vi "ResultsDB Select Record List.vi"() -> (0 "error out":errorcluster, 2 "Row Num List":string[](array[string]), 3 "Table Control":string[][](table))   [LabVIEW 2021, in "SQLite.lvclass"]
doc: "开始测试时根据条目自动创建条目条目，生产文件路径。\n#2020-6-8 13:25:45"
uses:
  SQLite.lvclass
  <vilib>/Utility/error.llb/Trim Whitespace.vi
  SQLite.lvclass/SQLite.ctl
  <userlib>/sushu/sushu.lvlib
  <userlib>/LabSQL/LabSQL.lvlib
  vi.lib_New/TopPath/TopPath.lvlib
panel:
  out "CMD":string
  out "number (0 to 1)":dbl
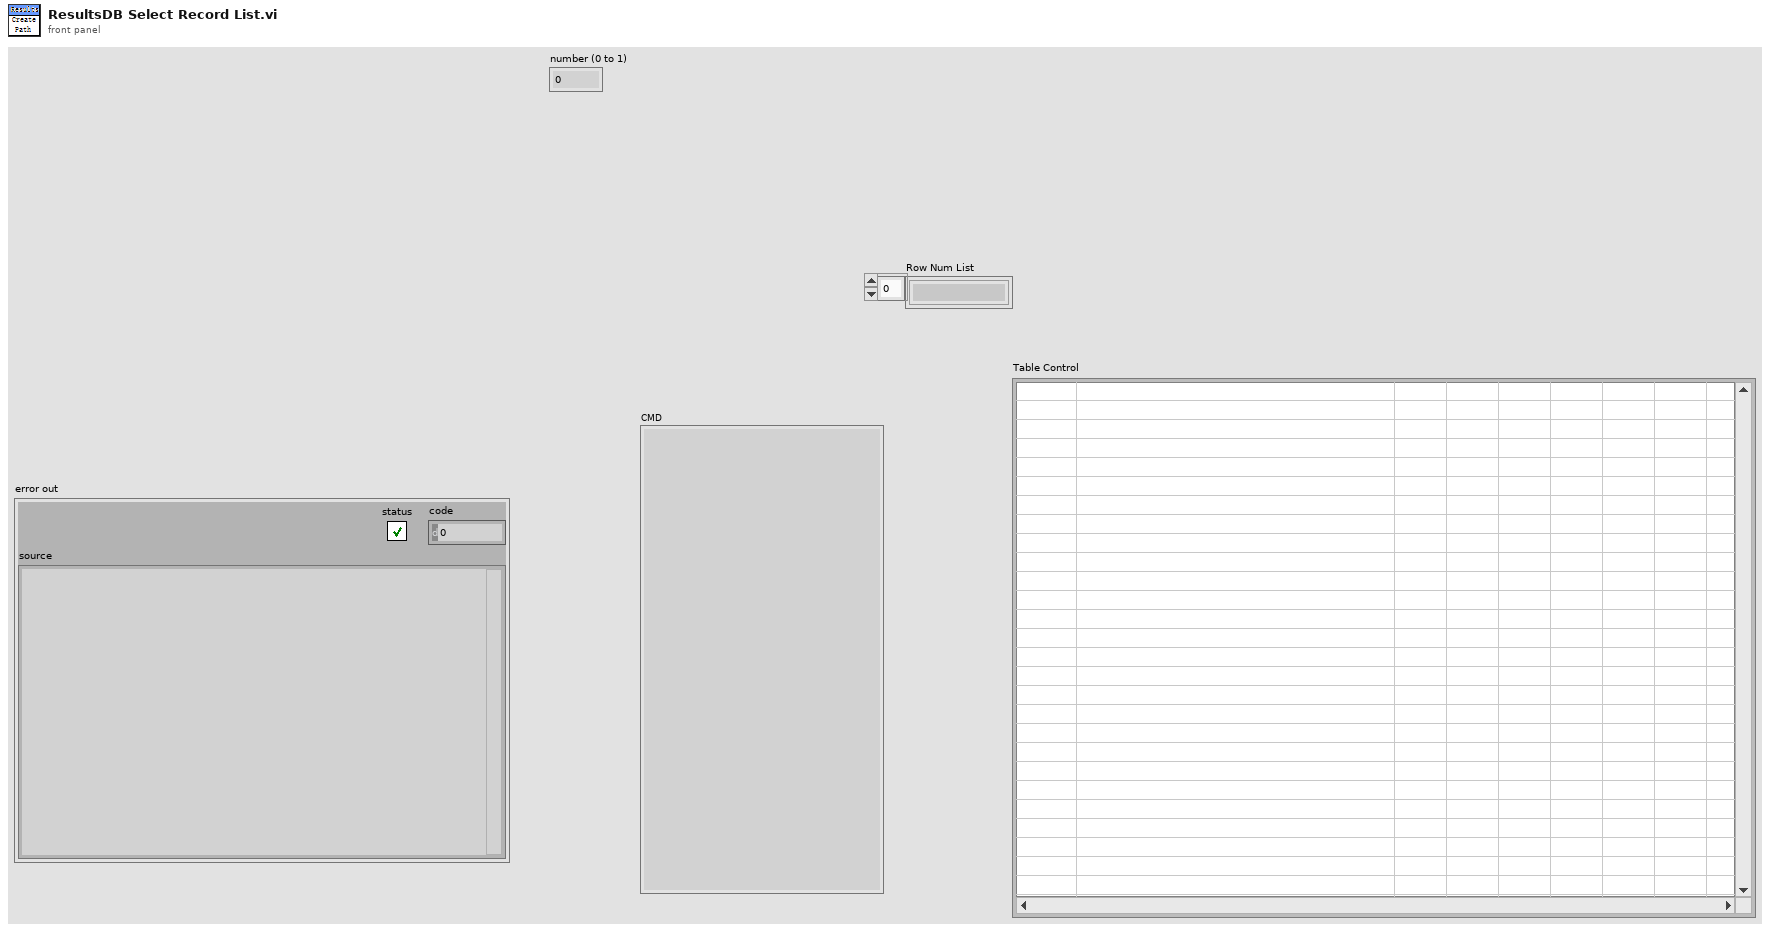
[diagram p1: front panel]
types:
  T1 = cluster{"Core":cluster{"Current VI Reference":refnum<vi>, "Close Panel on Exit?":bool}, "VI Name":string, "Row Numbers":string, "Update?":bool, "Results Folder path":path, "CMD":string, "RowNum":i32, "ResultFilePath":path, "InsertTimes":i32, "length":i32}
  T2 = enum16{"Other", "SQL2008", "SQLite", "Access", "MySQL"}
  T3 = typedef "TopPath.lvlib/Top Path.ctl" = cluster{"LV Source":path, "FilePath":path, "Data":path}
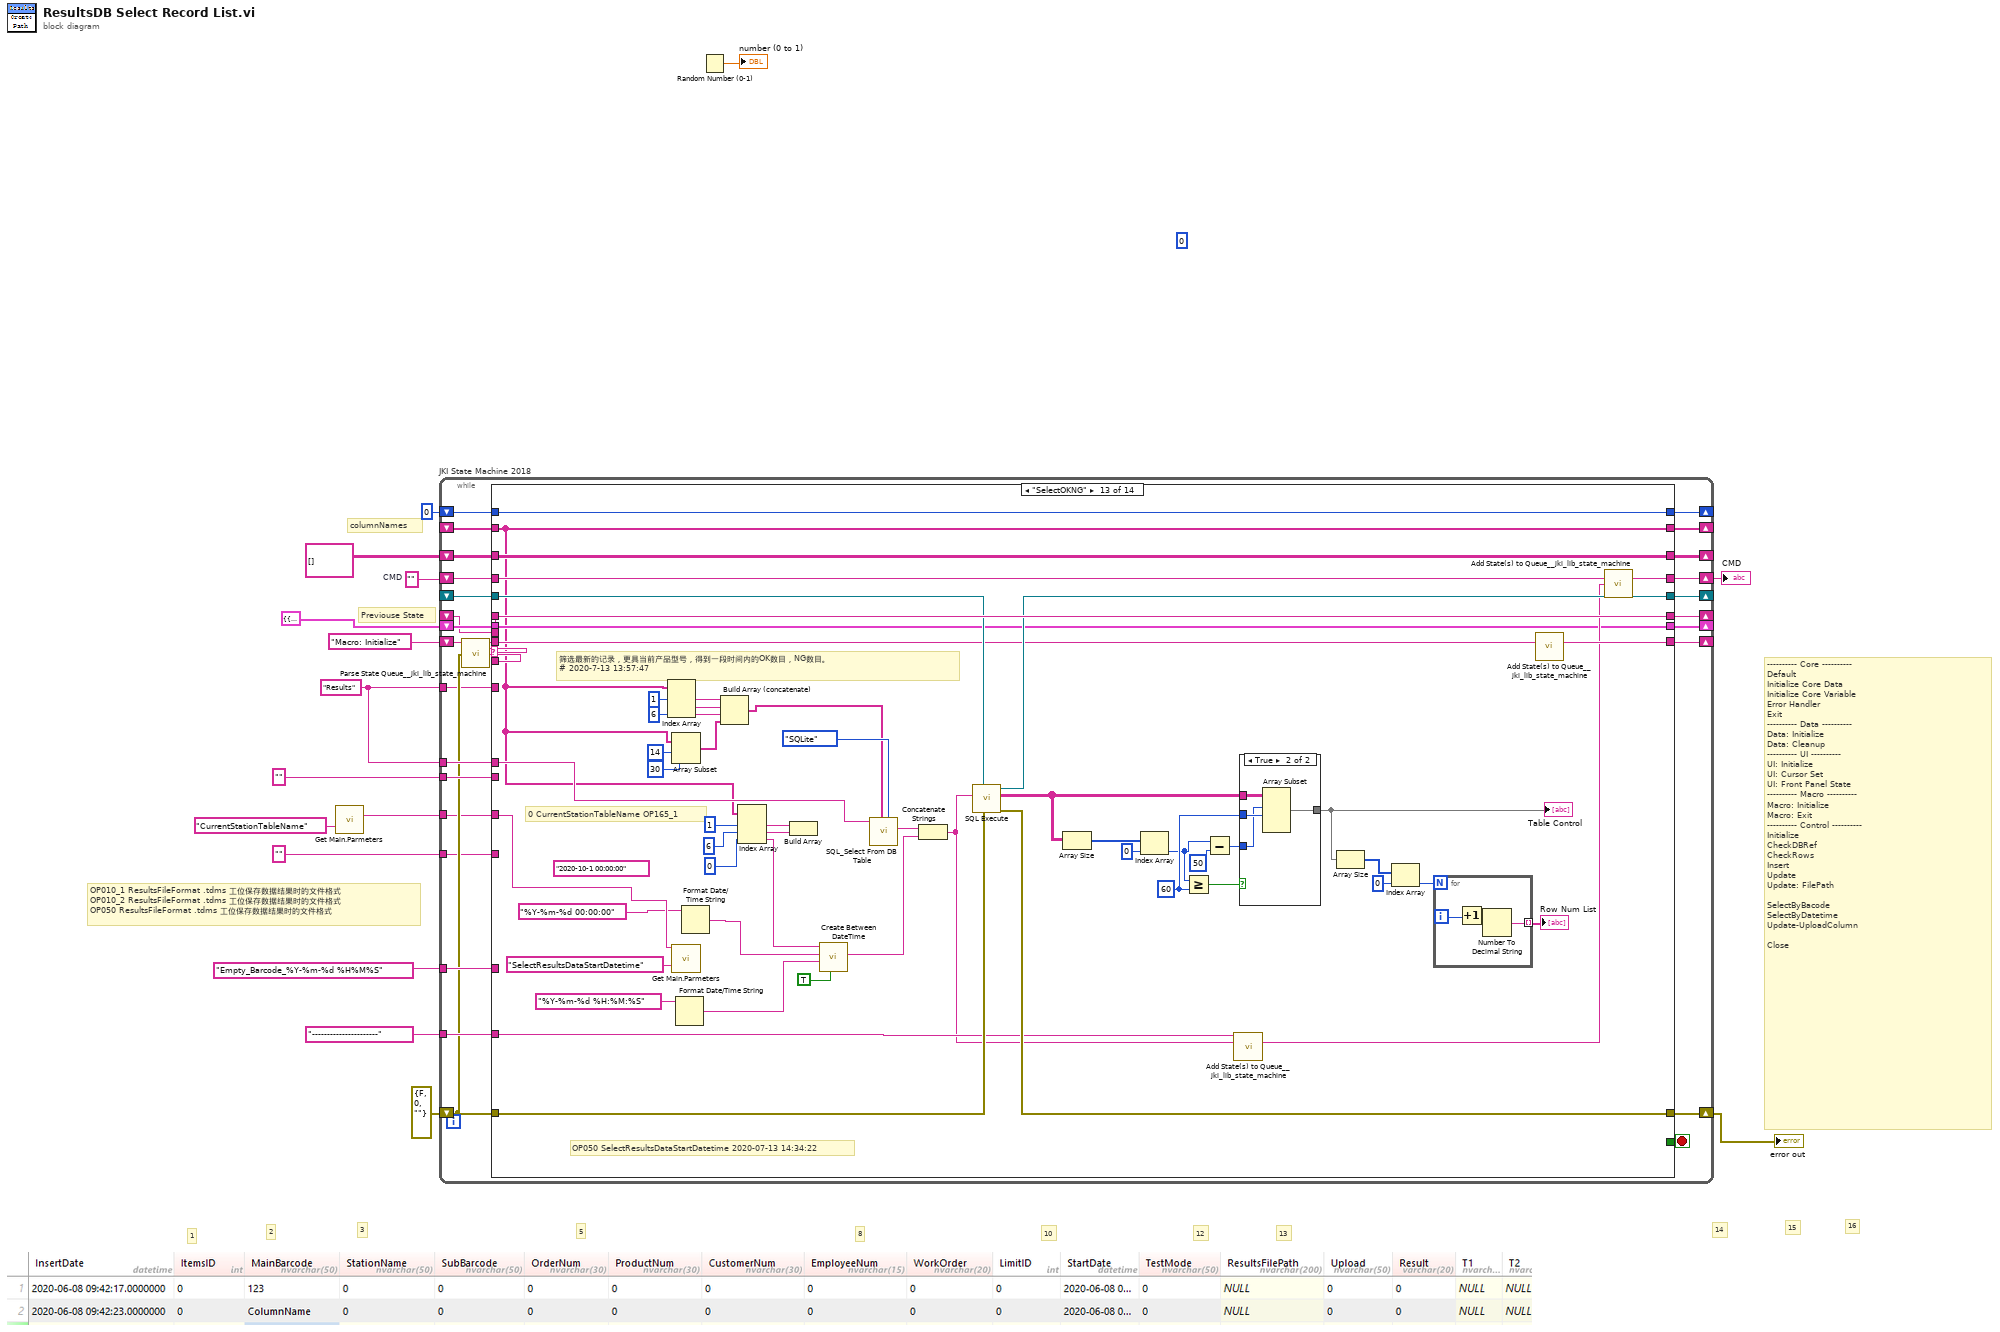
[diagram p0: block diagram]
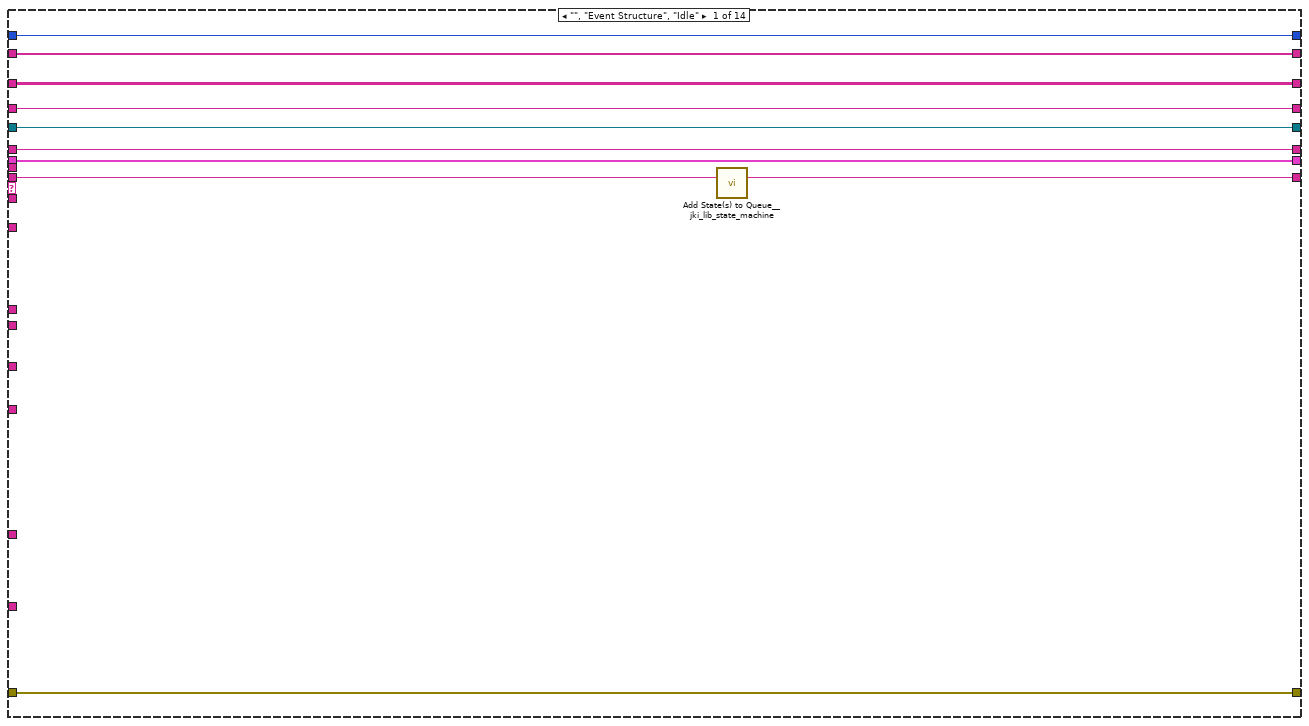
[diagram p2: hidden frame]
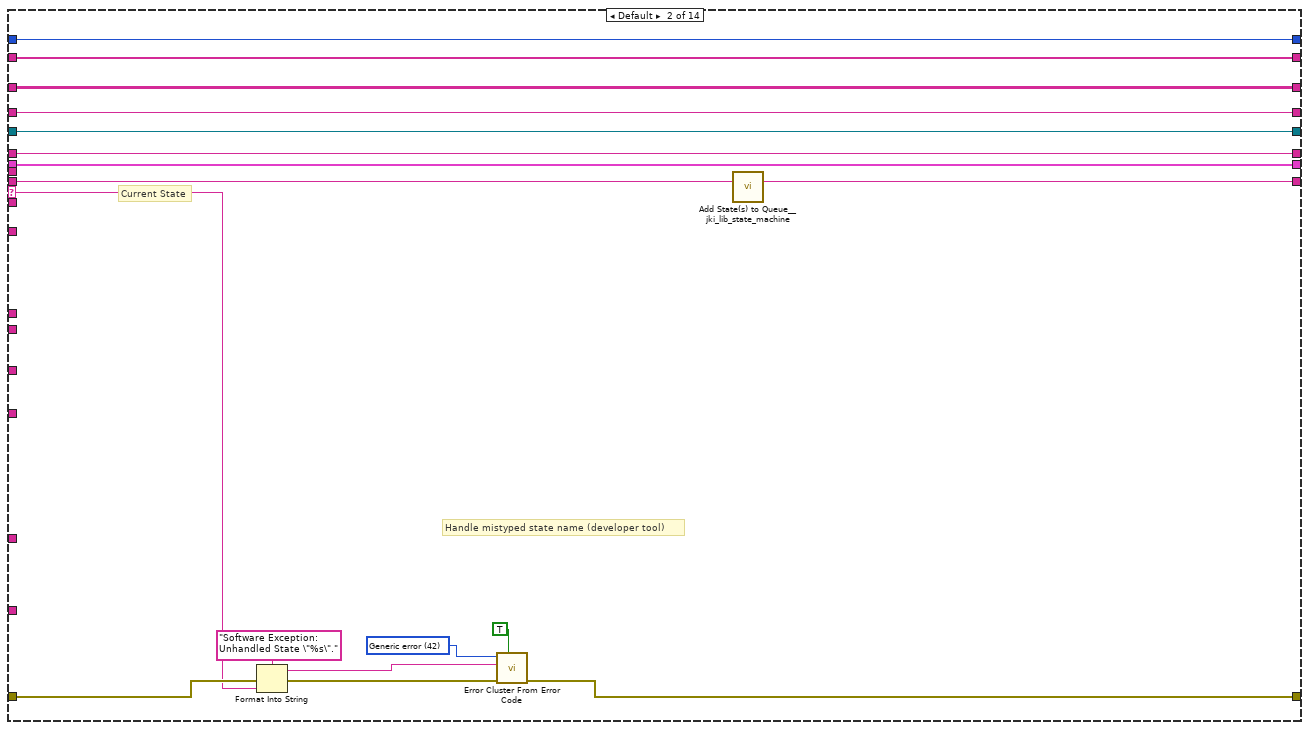
[diagram p3: hidden frame]
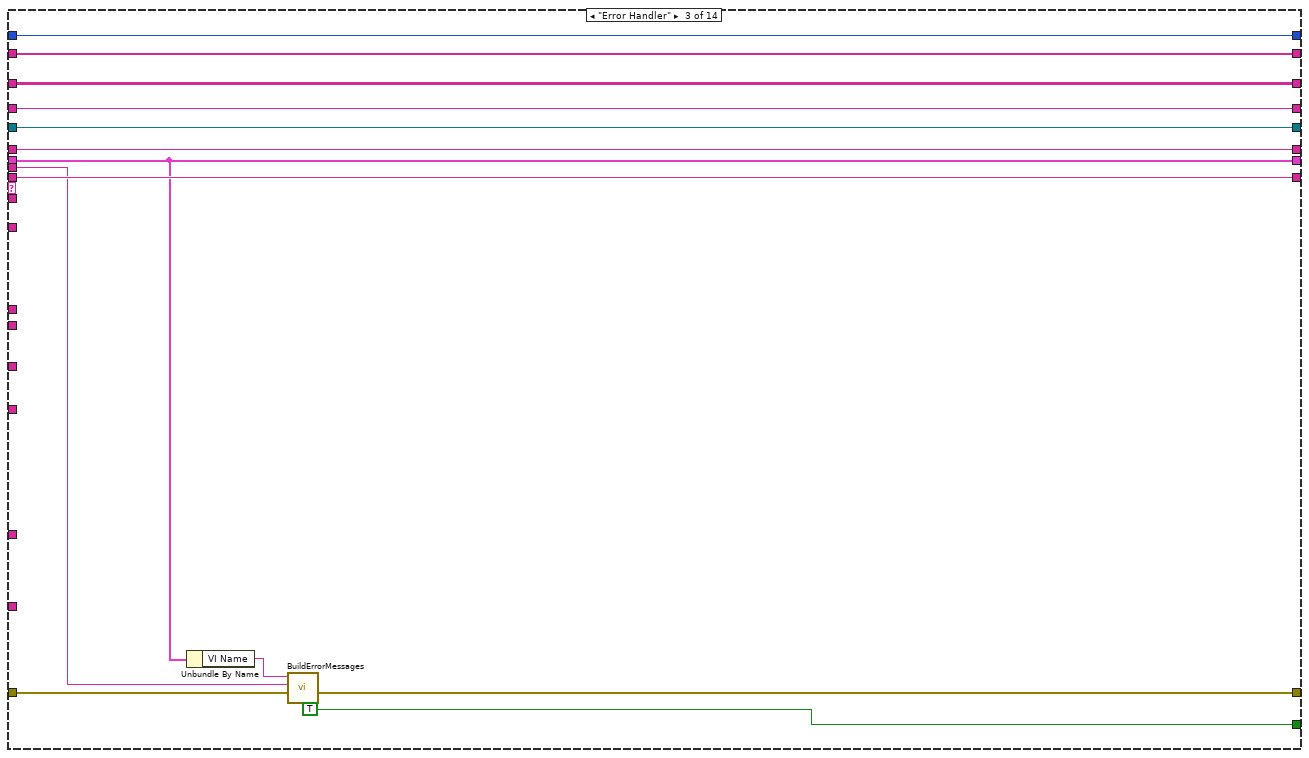
[diagram p4: hidden frame]
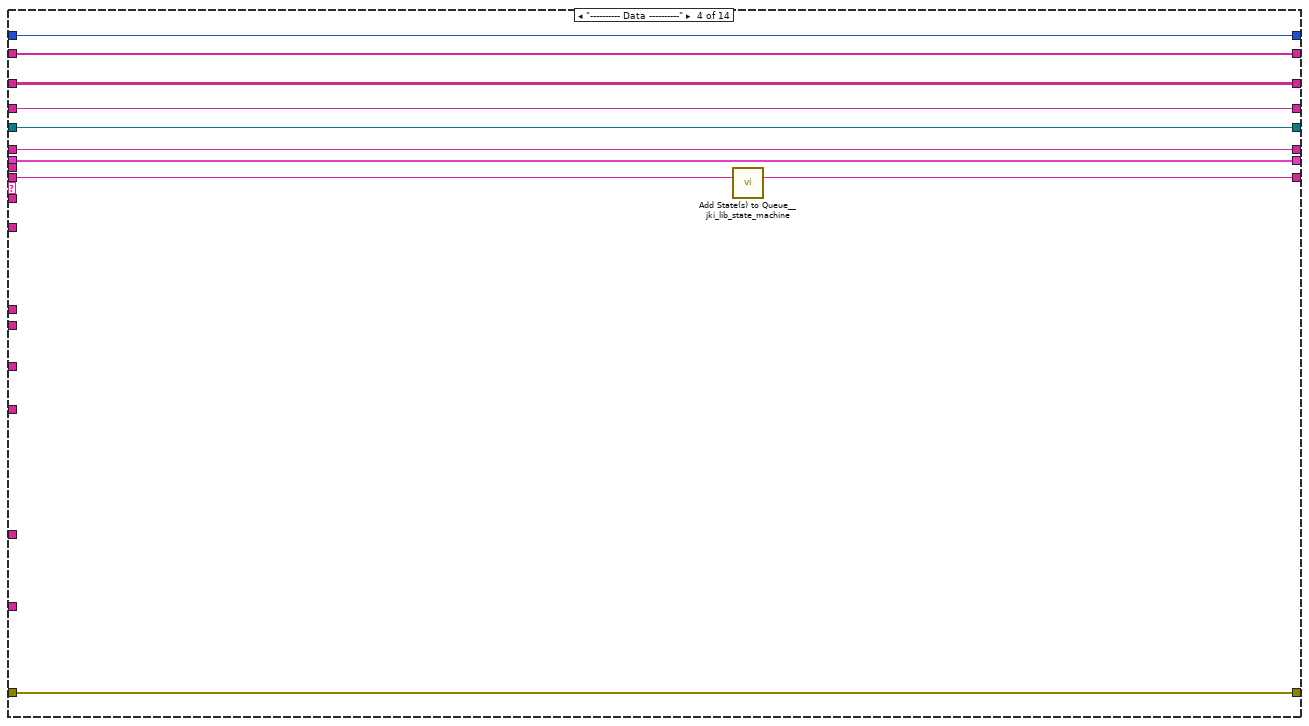
[diagram p5: hidden frame]
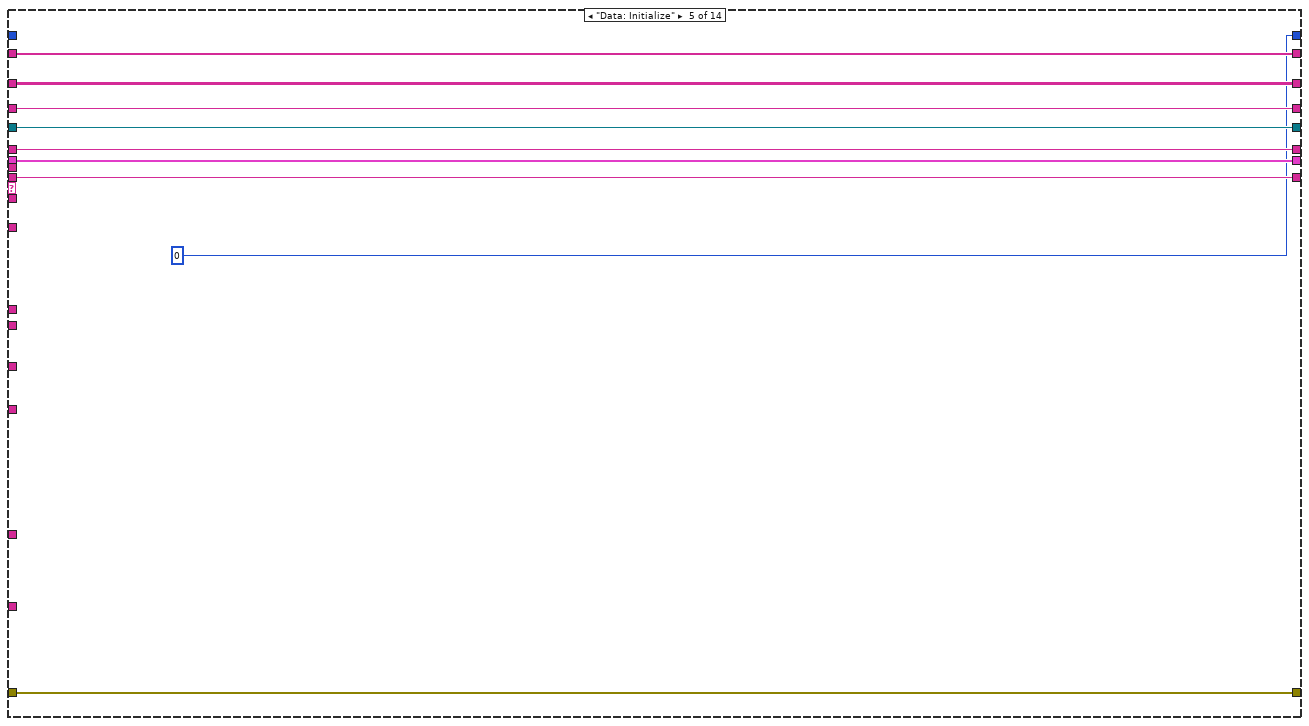
[diagram p6: hidden frame]
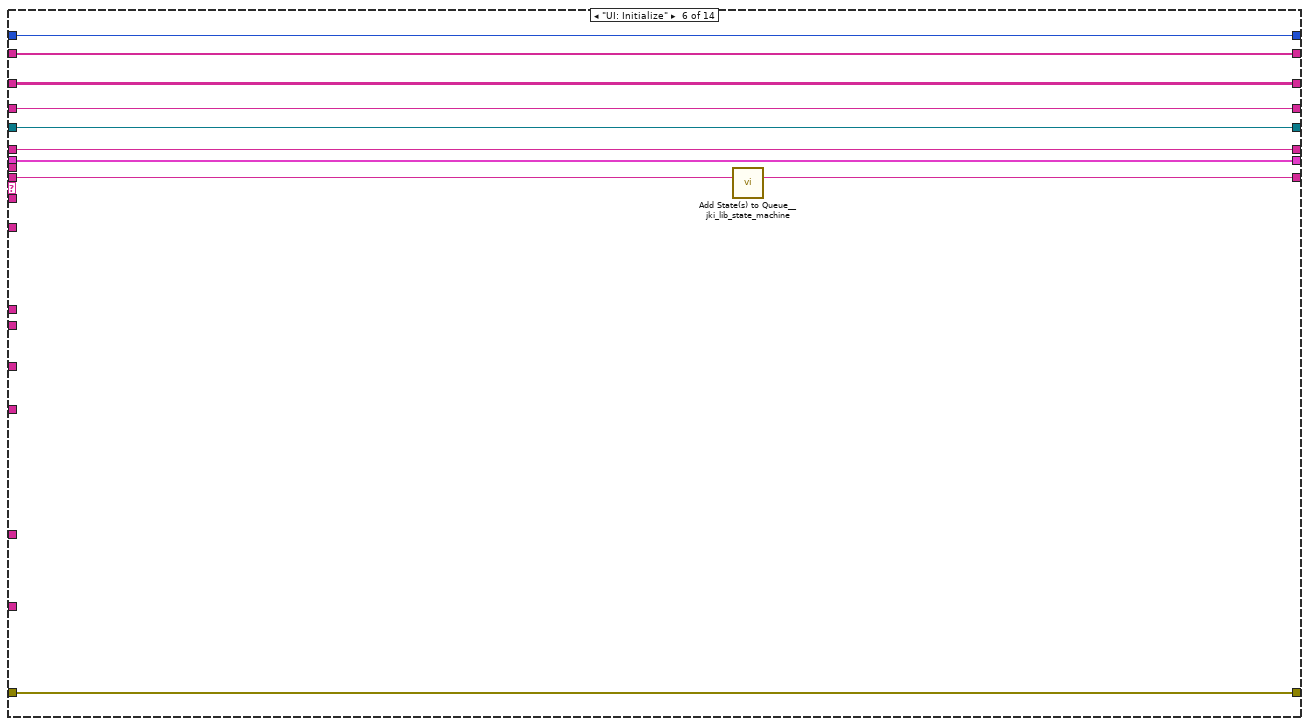
[diagram p7: hidden frame]
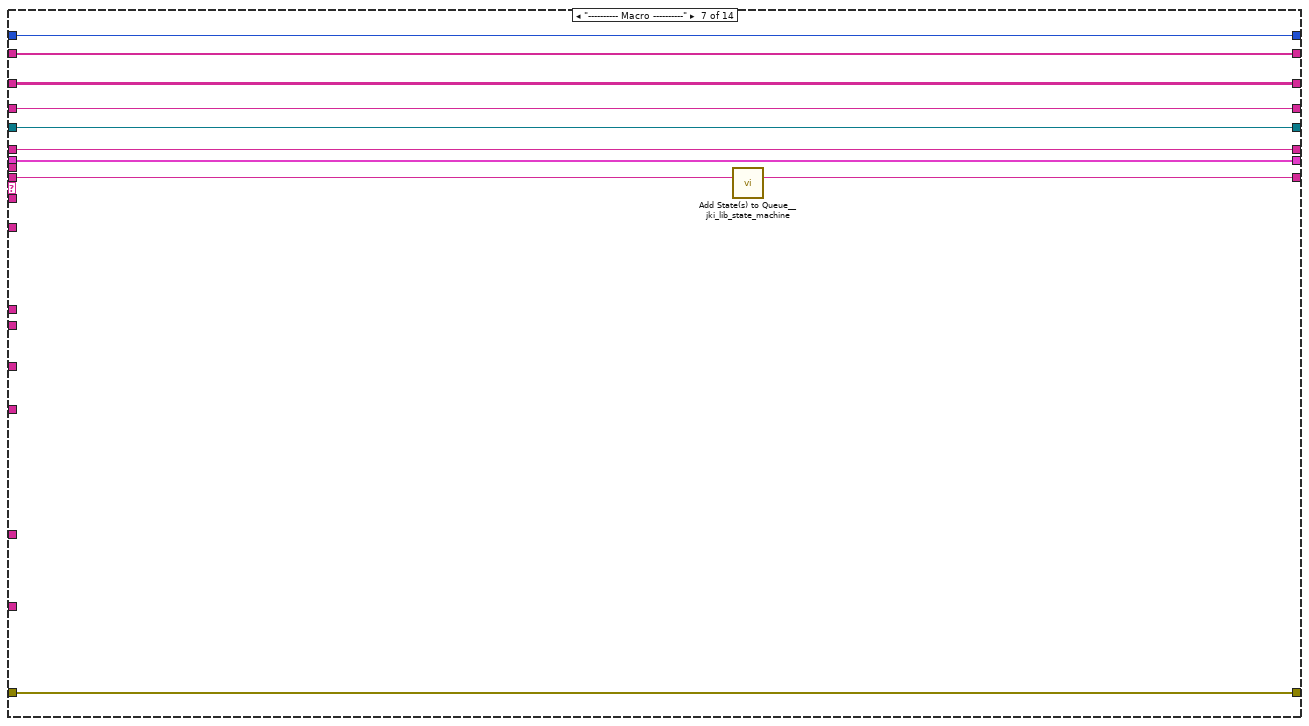
[diagram p8: hidden frame]
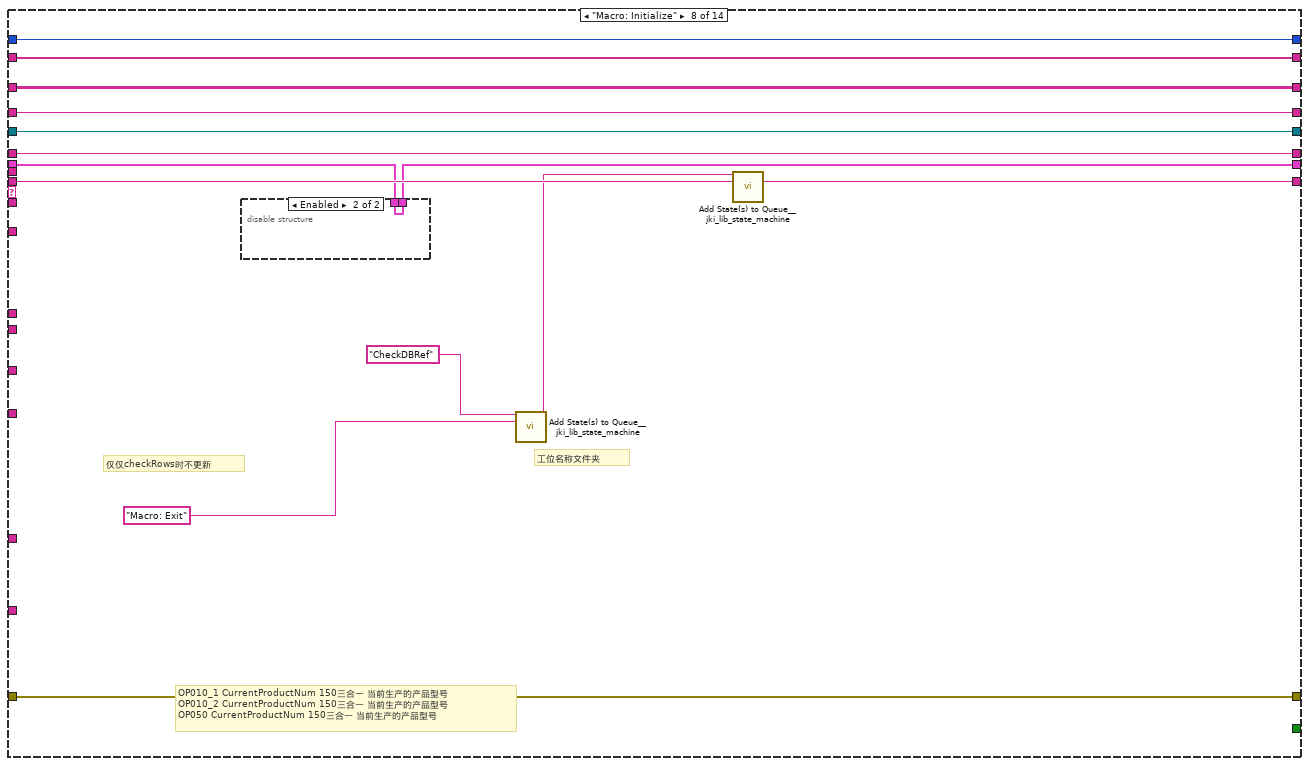
[diagram p9: hidden frame]
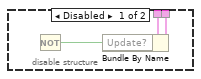
[diagram p10: hidden frame]
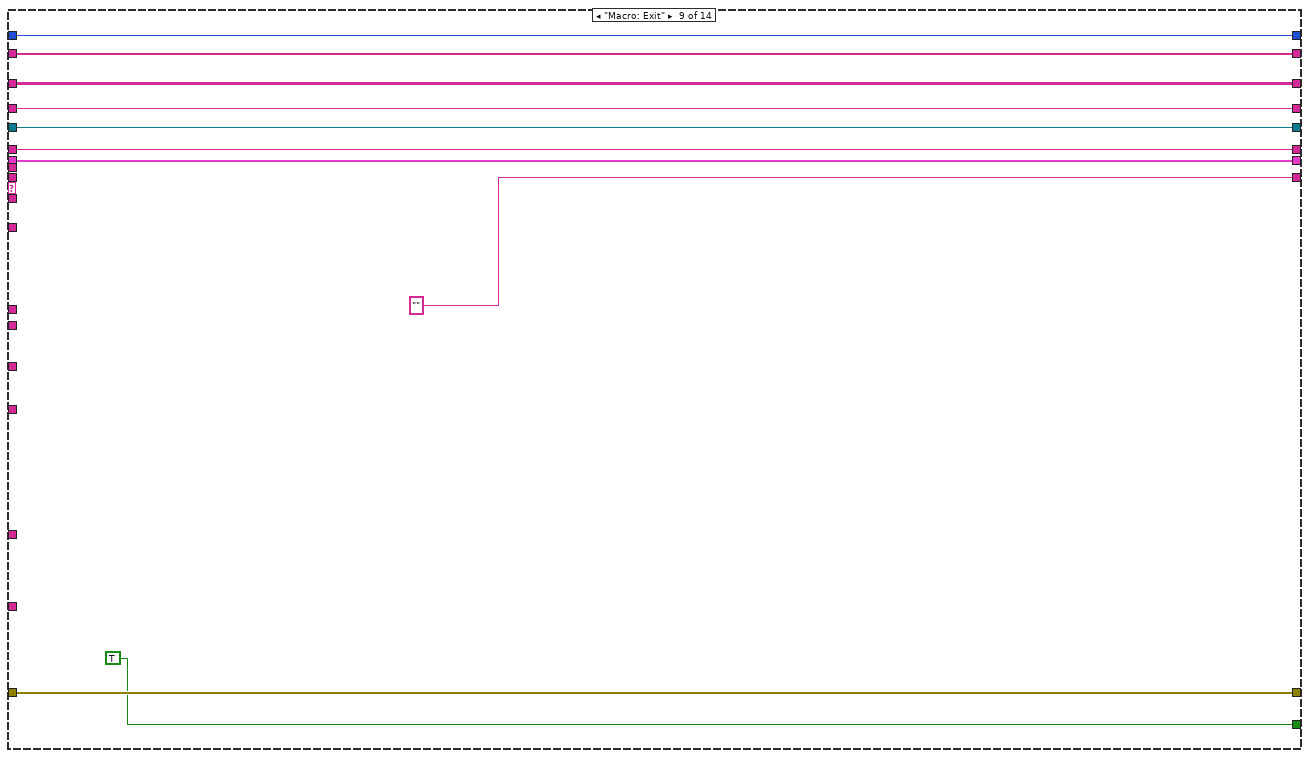
[diagram p11: hidden frame]
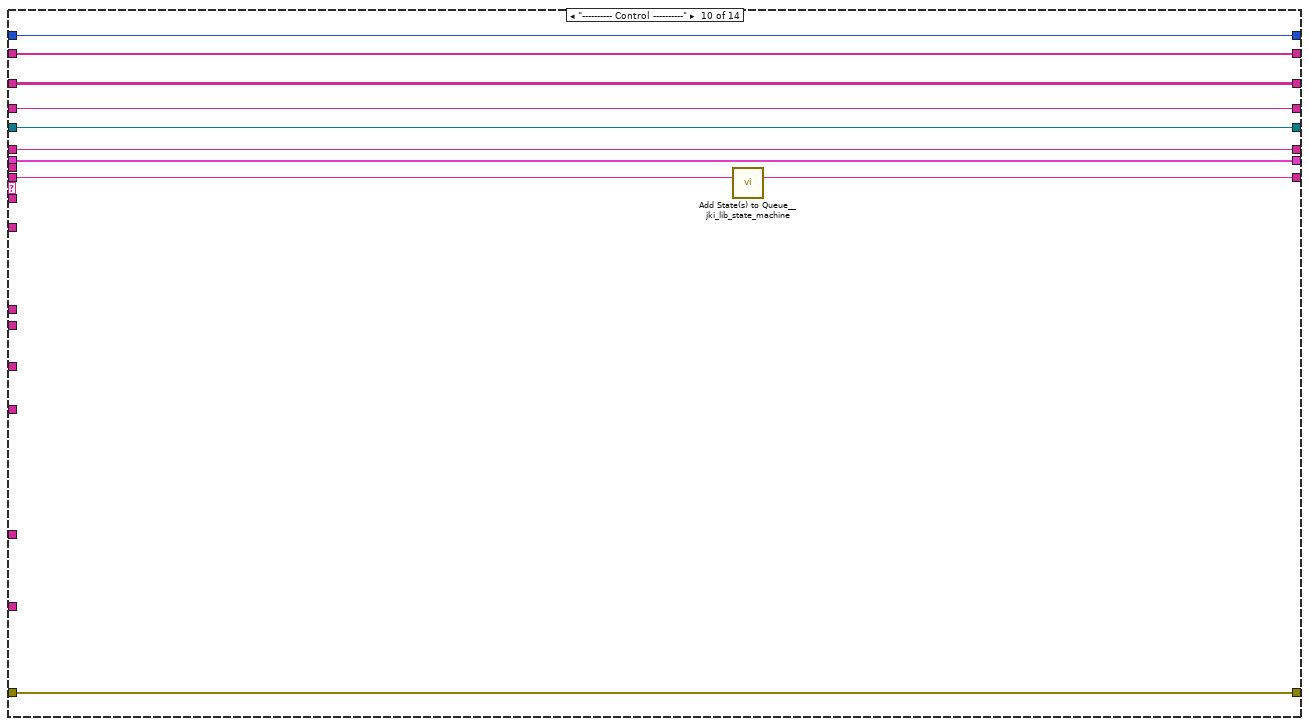
[diagram p12: hidden frame]
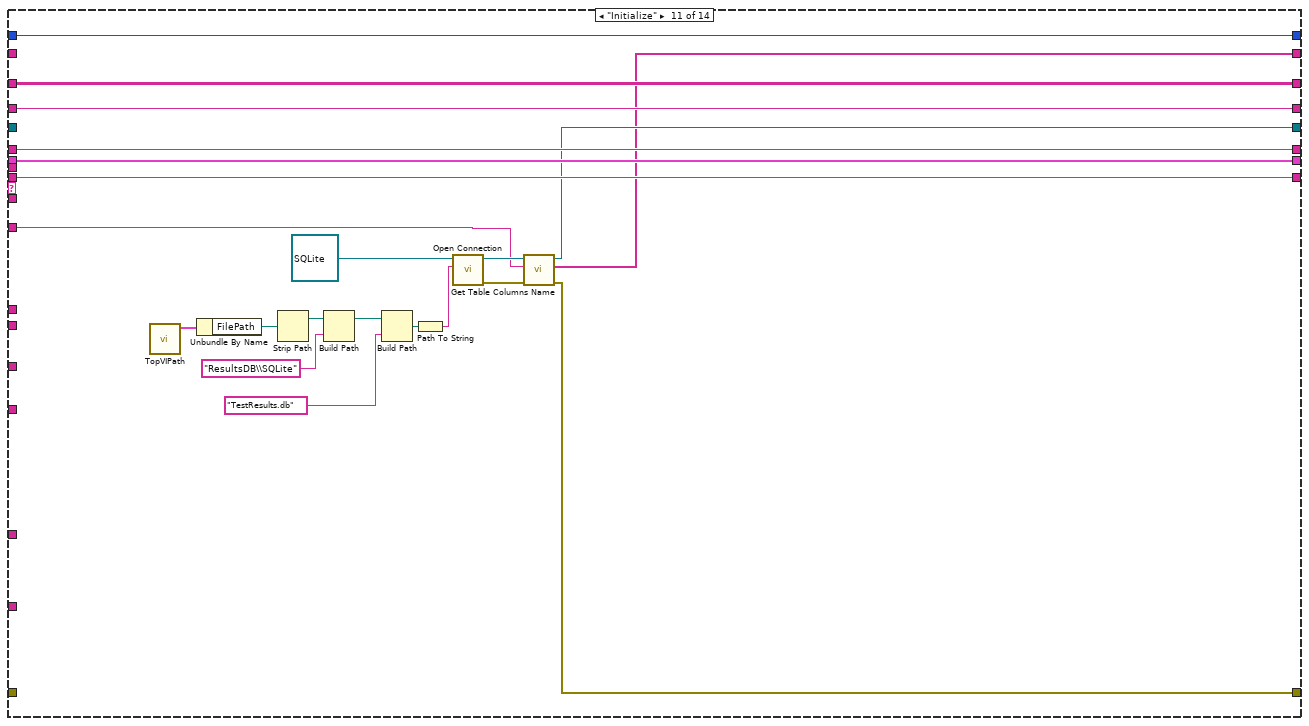
[diagram p13: hidden frame]
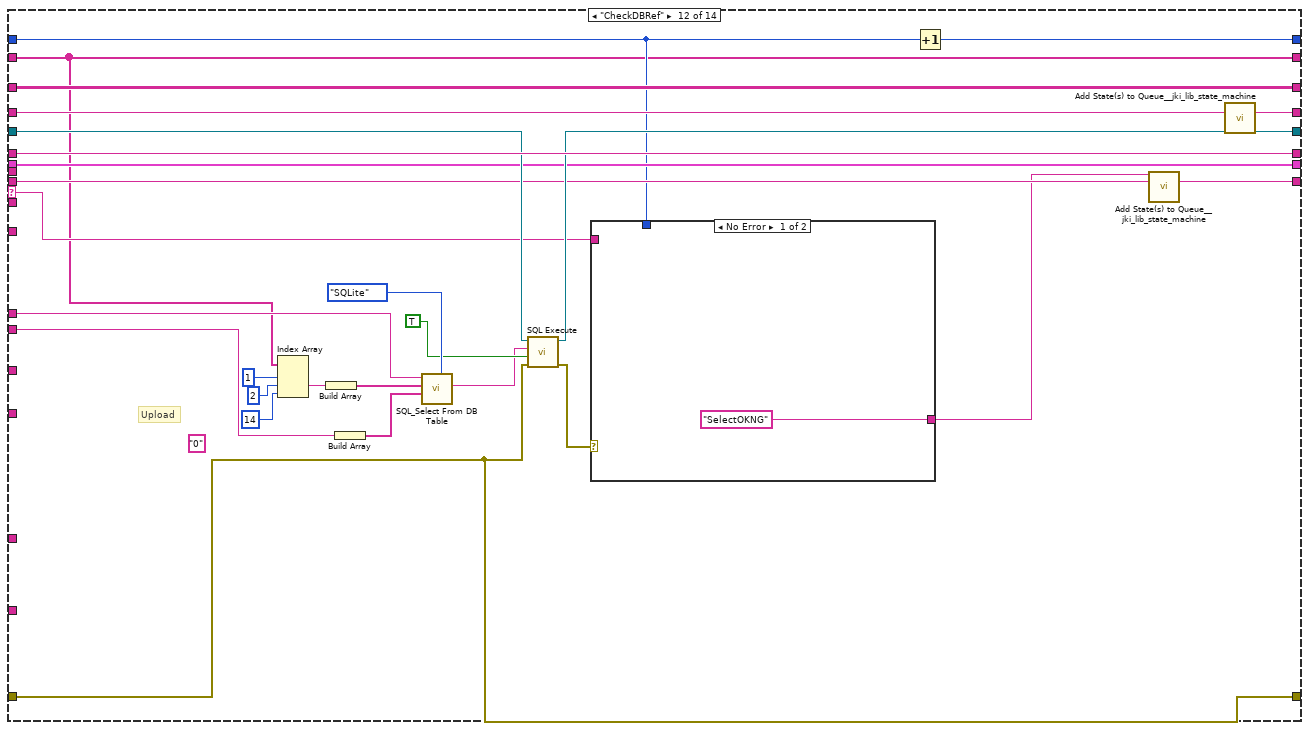
[diagram p14: hidden frame]
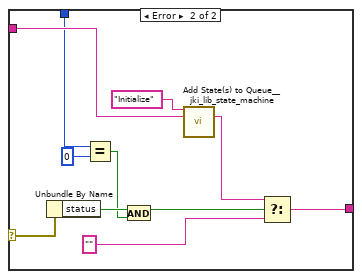
[diagram p15: hidden frame]
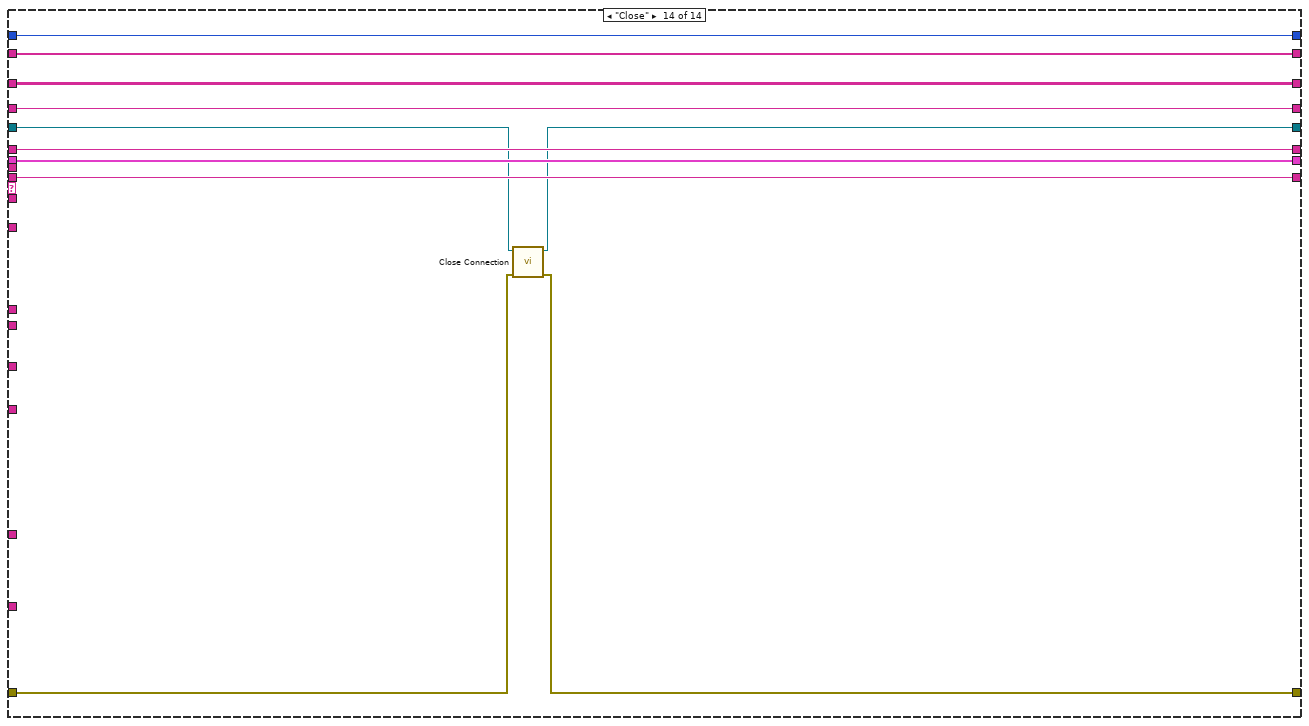
[diagram p17: hidden frame]
diagram:
  w7 = "Results" ("TableName")
  w9 = ""  # CMD
  (unwired) 0 ("index (row)")
  # "columnNames"
  # "OP010_1\tResultsFileFormat\t.tdms\t工位保存数据结果时的文件格式\nOP010_2\tResultsFileFormat\t.tdms\t工位保存数据结果时的文件格式\nOP050\tResultsFileFormat\t.tdms\t工位保存数据结果时的文件格式"
  # "16"
  # "15"
  # "14"
  # "13"
  # "12"
  # "10"
  # "8"
  # "5"
  # "3"
  # "2"
  # "1"
  # "Previouse State"
  # "---------- Core ----------\nDefault\nInitialize Core Data\nInitialize Core Variable\nError Handler\nExit\n---------- Data ----------\nData: Initialize\nData: Cleanup\n---------- UI ----------\nUI: Initialize\nUI: Cursor Set\nUI: Front Panel State\n---------- Macro ----------\nMacro: Initialize\nMacro: Exit\n---------- Control ----------\nInitialize\nCheckDBRef\nCheckRows\nInsert\nUpdate\nUpdate: FilePath\n\nSelectByBacode\nSelectByDatetime\nUpdate-UploadColumn\n\nClose"
  n1 = call "Get Main.Parmeters.vi"("VariableName"="CurrentStationTableName") -> ("Value"=w1:string)  [unwired: 7 in, 7 out]
  n2 = while "JKI State Machine 2018" {
    shift-right: [w39] -> _
    shift-left: T1 {"Core"={"Current VI Reference"=refnum, "Close Panel on Exit?"=FALSE}, "VI Name"="", "Row Numbers"="", "Update?"=FALSE, "Results Folder path"=path "", "CMD"="", "RowNum"=0, "ResultFilePath"=path "", "InsertTimes"=0, "length"=3} ("Data") -> [w38]
    shift-right: [w42] -> w4
    shift-left: errorcluster {"status"=FALSE, "code"=0, "source"=""} ("error out") -> [w24]
    shift-right: [w41] -> _
    shift-left: "Macro: Initialize" -> [w43]
    shift-right: [w36] -> _
    shift-left: _ -> [w37]
    shift-right: [w34] -> _
    shift-left: _ -> [w33]
    tunnel: "" ("MainBarcode") -> [w32]
    tunnel: w7 -> [w31]
    tunnel: "Empty_Barcode_%Y-%m-%d %H%M%S" ("time format string (%c)") -> [w30]
    shift-right: [w29] -> w3
    shift-left: w9 -> [w28]
    tunnel: "----------------------" ("State(s) in (\"\")") -> [w27]
    shift-right: [w25] -> _
    shift-left: string[][] [] ("Table Control") -> [w26]
    tunnel: "" ("ItemsID") -> [w23]
    tunnel: w7 -> [w22]
    shift-right: [w21] -> _
    shift-left: _ -> [w20]
    shift-right: [w18] -> _
    shift-left: 0 -> [w19]
    tunnel: w1 -> [w17]
    stop <- w40 stop-if-true
    n3 = call <vilib>:"Parse State Queue__jki_lib_state_machine.vi"("State Queue"=w43, "Error In (no error)"=w24) -> ("Remaining States"=w45:string, "Current State"=w35:string, "Arguments"=w44:string)  [unwired: 10 in, 1 out]
    n4 = case shown="\"SelectOKNG\"" w35 {
      selector: w35 -> [_ w62 _ _ _ _ _ _ _ _ _ w189 _ _]
      tunnel: w45 -> [w55 w66 w84 w95 w101 w114 w124 w138 _ w162 w183 w199 w269 w296]
      tunnel: w44 -> [_ _ _ _ _ _ _ _ _ _ _ _ _ _]
      tunnel: w38 -> [w52 w64 w81 w92 w102 w112 w121 w133 w151 w159 w182 w195 w249 w295]
      tunnel: [w53 w68 w77 w93 w104 w111 w122 w134 w152 w160 w166 w188 w267 w286] -> w42
      tunnel: w24 -> [w53 w67 w78 w93 w104 w111 w122 w134 w152 w160 _ w188 w268 w287]
      tunnel: [w54 w65 w84 w94 w101 w113 w123 w137 "" w161 w183 w200 w270 w296] -> w41
      tunnel: [_ _ TRUE _ _ _ _ _ TRUE _ _ _ _ _] -> w40
      tunnel: [w52 w64 w81 w92 w102 w112 w121 w128 w151 w159 w182 w195 w249 w295] -> w39
      tunnel: w37 -> [w51 w61 w83 w91 w103 w110 w120 w136 w150 w158 _ w203 w272 w289]
      tunnel: [w51 w61 w83 w91 w103 w110 w120 w136 w150 w158 w167 w202 w271 w288] -> w36
      tunnel: w35 -> [w50 w60 w82 w90 w100 w109 w119 w135 w148 w157 w181 w210 w277 w294]
      tunnel: [w50 w60 w82 w90 w100 w109 w119 w135 w148 w157 w181 w210 w277 w294] -> w34
      tunnel: w33 -> [_ _ w79 _ _ _ _ _ _ _ _ _ _ _]
      tunnel: w32 -> [_ _ _ _ _ _ _ _ _ _ _ w204 _ _]
      tunnel: w31 -> [_ _ _ _ _ _ _ _ _ _ _ w205 w273 _]
      tunnel: w30 -> [_ _ _ _ _ _ _ _ _ _ _ _ _ _]
      tunnel: w28 -> [w49 w59 w76 w89 w99 w108 w118 w130 w146 w156 w180 w197 w265 w293]
      tunnel: [w49 w59 w76 w89 w99 w108 w118 w130 w146 w156 w180 w198 w266 w293] -> w29
      tunnel: w27 -> [_ _ _ _ _ _ _ _ _ _ _ _ w262 _]
      tunnel: w26 -> [w48 w58 w75 w88 w98 w107 w117 w129 w145 w155 w179 w191 w250 w292]
      tunnel: [w48 w58 w75 w88 w98 w107 w117 w129 w145 w155 w179 w191 w250 w292] -> w25
      tunnel: w23 -> [_ _ _ _ _ _ _ _ _ _ _ _ _ _]
      tunnel: w22 -> [_ _ _ _ _ _ _ _ _ _ w165 _ _ _]
      tunnel: w20 -> [w47 w57 w74 w87 w97 w106 w116 w127 w144 w154 _ w184 w242 w291]
      tunnel: [w47 w57 w74 w87 w97 w106 w116 w127 w144 w154 w164 w184 w242 w291] -> w21
      tunnel: w19 -> [w46 w56 w73 w86 _ w105 w115 w125 w143 w153 w163 w185 w255 w290]
      tunnel: [w46 w56 w73 w86 0 w105 w115 w125 w143 w153 w163 w186 w255 w290] -> w18
      tunnel: w17 -> [_ _ _ _ _ _ _ _ _ _ _ _ w240 _]
      frame "", "Event Structure", "Idle" {
        n5 = call <vilib>:"Add State(s) to Queue__jki_lib_state_machine.vi"("State(s) in (\"\")"=w55) -> ("States Out"=w54:string)  [unwired: 14 in]
      }
      frame Default {
        w71 = 42 items=["No error", "Argument error", "Memory is full", "Out of zone", "End of file", "File already open", "Generic file I/O error", "File not found", "File permission error", "Disk is full", "Duplicate path", "Too many files open", "System feature not enabled", "Resource file not found", "Cannot add resource", "Resource not found", "Image not found", "Image memory error", "Pen does not exist", "Config type invalid", "Config token not found", "Config parse error", "Config memory error", "Bad external code format", "Bad external code offset", "External code not present", "Null window", "Destroy window error", "Null menu", "Print aborted", "Bad print record", "Print driver error", "Windows error during printing", "Memory error during printing", "Print dialog error", "Generic print error", "Invalid device refnum", "Device not found", "Device parameter error", "Device unit error", "Cannot open device", "Device call aborted", "Generic error", "Cancelled by user", "Object ID too low", "Object ID too high", "Object not in heap", "Unknown heap", "Unknown object (invalid DefProc)", "Unknown object (DefProc not in table)", "Message out of range", "Invalid (null) method", "Unknown message", "Manager call not supported", "Bad address", "Network operation in progress", "Network operation timed out", "Connection is busy", "Network attribute not supported", "Network error", "Address in use", "System out of memory", "Connection aborted", "Connection refused", "Not connected", "Already connected", "Connection closed", "Initialization error (interapplication manager)", "Bad occurrence", "Wait on unbound occurrence handler", "Occurrence queue overflow", "Datalog type conflict", "Unused", "Unrecognized type (interapplication manager)", "Memory corrupt", "Failed to make temporary DLL", "Old CIN version", "Drag socket not found", "Failed to load drop-object", "Failed to register OLE object", "Failed to release OLE object", "Format specifier type mismatch", "Unknown format specifier", "Too few format specifiers", "Too many format specifiers", "Scan failed", "Newer CIN version", "Error converting to variant", "Runtime menu error", "Password tampered", "Variant attribute not found", "Incompatible variant data type", "Event data is not available", "Event Store is not present", "Occurrence is not found", "Event Queue is not created", "Event info is not available", "Refnum passed is NULL", "Error retrieving Class GUID", "Error retrieving CoClass GUID", "Error retrieving TypeLib GUID.", "Bad built application magic bytes.", "Specific driver is different from the specific driver associated with the Logical Name.", "There is no session opened to the class driver.", "Max Error", "MAX - Error with config objects", "MAX - Error loading configuration", "MAX - Group not supported"]
        # "Current State"
        # "Handle mistyped state name (developer tool)"
        n6 = Format Into String(format string="Software Exception: Unhandled State \"%s\"." ("message"), error in=w67, w62) -> (resulting string=w70:string, error out=w69:errorcluster)  [unwired: 1 in]
        n7 = call <vilib>:"Error Cluster From Error Code.vi"("show call chain? (False)"=TRUE, "error in (no error)"=w69, "error message (\"\")"=w70, "error code (0)"=w71) -> ("error out"=w68:errorcluster)  [unwired: 5 in]
        n8 = call <vilib>:"Add State(s) to Queue__jki_lib_state_machine.vi"("State(s) in (\"\")"=w66) -> ("States Out"=w65:string)  [unwired: 14 in]
      }
      frame "Error Handler" {
        n9 = Unbundle By Name(w81) -> ("VI Name"=w80:string)
        n10 = call <userlib>:"BuildErrorMessages.vi"("error in"=w78, "ErrorCase"=w79, "VI Name"=w80) -> ("error out (no error)"=w77:errorcluster)  [unwired: 6 in, 2 out]
      }
      frame "---------- Data ----------" {
        n11 = call <vilib>:"Add State(s) to Queue__jki_lib_state_machine.vi"("State(s) in (\"\")"=w95) -> ("States Out"=w94:string)  [unwired: 14 in]
      }
      frame "Data: Initialize" {
      }
      frame "UI: Initialize" {
        n12 = call <vilib>:"Add State(s) to Queue__jki_lib_state_machine.vi"("State(s) in (\"\")"=w114) -> ("States Out"=w113:string)  [unwired: 14 in]
      }
      frame "---------- Macro ----------" {
        n13 = call <vilib>:"Add State(s) to Queue__jki_lib_state_machine.vi"("State(s) in (\"\")"=w124) -> ("States Out"=w123:string)  [unwired: 14 in]
      }
      frame "Macro: Initialize" {
        # "OP010_1\tCurrentProductNum\t150三合一\t当前生产的产品型号\nOP010_2\tCurrentProductNum\t150三合一\t当前生产的产品型号\nOP050\tCurrentProductNum\t150三合一\t当前生产的产品型号"
        # "工位名称文件夹"
        # "仅仅checkRows时不更新"
        n14 = disable-structure shown="Enabled" {
          disable-tunnel: w133 -> [w141 w142]
          disable-tunnel: [w140 w142] -> w128
          frame Disabled {
            n15 = Not() -> (.not. x?=w139:bool)  [unwired: 1 in]
            n16 = Bundle By Name(cluster=w141, "Update?"=w139) -> (w140:T1)
          }
          frame Enabled {
          }
        }
        n17 = call <vilib>:"Add State(s) to Queue__jki_lib_state_machine.vi"("State(s) in Front (\"\")"="CheckDBRef" ("State(s) in Front (\"\")"), "State(s) in (\"\")"="Macro: Exit") -> ("States Out"=w132:string)  [unwired: 13 in]
        n18 = call <vilib>:"Add State(s) to Queue__jki_lib_state_machine.vi"("State(s) in Front (\"\")"=w132, "State(s) in (\"\")"=w138) -> ("States Out"=w137:string)  [unwired: 13 in]
      }
      frame "Macro: Exit" {
      }
      frame "---------- Control ----------" {
        n19 = call <vilib>:"Add State(s) to Queue__jki_lib_state_machine.vi"("State(s) in (\"\")"=w162) -> ("States Out"=w161:string)  [unwired: 14 in]
      }
      frame "Initialize" {
        n20 = call "TopVIPath.vi"() -> ("TopPath"=w178:T3)  [unwired: 10 in, 1 out]
        n21 = Unbundle By Name(w178) -> ("FilePath"=w168:path)
        n22 = Strip Path(path=w168) -> (stripped path=w169:path)  [unwired: 1 out]
        n23 = Build Path(base path=w169, name or relative path="ResultsDB\\SQLite") -> (appended path=w171:path)
        n24 = Build Path(base path=w171, name or relative path="TestResults.db") -> (appended path=w173:path)
        n25 = Path To String(path=w173) -> (string=w174:string)
        n26 = call-dynamic "Open Connection.vi"("ConnectionString"=w174, "HostDB in"=refnum<class "SQLite.lvclass"> refnum ("SQLite.lvclass")) -> ("error out"=w176:errorcluster, "HostDB out"=w175:refnum<class "SQLite.lvclass">)  [unwired: 8 in]
        n27 = call-dynamic "Get Table Columns Name.vi"("error in (no error)"=w176, "TableName"=w165, "HostDB in"=w175) -> ("error out"=w166:errorcluster, "Table_ColunmsList"=w164:string[], "HostDB out"=w167:refnum<class "SQLite.lvclass">)  [unwired: 4 in, 2 out]
      }
      frame "CheckDBRef" {
        (unwired) "0" ("State(s) in (\"\")")
        # "Upload"
        n28 = Index Array(array=w184, index #1=1 ("index"), index #2=2 ("index"), index #3=14 ("index")) -> (element #2=w193:string)  [unwired: 2 out]
        n29 = Build Array(w193) -> (w208:string[])
        n30 = Build Array(w204) -> (w207:string[])
        n31 = call <userlib>:"SQL_Select From DB Table.vi"("DB Type"=T2."SQLite", "ColumnsValue"=w207, "ColumnsNameList"=w208, "TableName"=w205) -> ("Select SQL CMD"=w196:string)  [unwired: 7 in]
        n32 = call-dynamic "SQL Execute.vi"("error in (no error)"=w188, "Return Data (T)"=TRUE, "Command Text"=w196, "HostDB in"=w203) -> ("error out"=w190:errorcluster, "HostDB out"=w202:refnum<class "SQLite.lvclass">)  [unwired: 3 in, 3 out]
        n33 = case shown="No Error" w190 {
          selector: w190 -> [_ w218]
          tunnel: w189 -> [_ w219]
          tunnel: ["SelectOKNG" ("resulting string") w217] -> w187
          tunnel: w185 -> [_ w214]
          frame No Error {
          }
          frame Error {
            n34 = Unbundle By Name(w218) -> ("status"=w216:bool)
            n35 = Equal?(x=w214, y=0) -> (x = y?=w212:bool)
            n36 = And(x=w216, y=w212) -> (x .and. y?=w215:bool)
            n37 = call <vilib>:"Add State(s) to Queue__jki_lib_state_machine.vi"("State(s) in Front (\"\")"="Initialize" ("Remaining States"), "State(s) in (\"\")"=w219) -> ("States Out"=w220:string)  [unwired: 13 in]
            n38 = Select(t=w220, s=w215, f="") -> (s? t:f=w217:string)
          }
        }
        n39 = Increment(x=w185) -> (x+1=w186:i32)
        n40 = call <vilib>:"Add State(s) to Queue__jki_lib_state_machine.vi"("State(s) in Front (\"\")"=w187, "State(s) in (\"\")"=w199) -> ("States Out"=w200:string)  [unwired: 13 in]
        n41 = call <vilib>:"Add State(s) to Queue__jki_lib_state_machine.vi"("State(s) in (\"\")"=w197) -> ("States Out"=w198:string)  [unwired: 14 in]
      }
      frame "SelectOKNG" {
        w233 = 60 ("y")
        (unwired) "2020-10-1 00:00:00" ("time format string (%c)")
        # "0\tCurrentStationTableName\tOP165_1"
        # "OP050\tSelectResultsDataStartDatetime\t2020-07-13 14:34:22"
        # "筛选最新的记录，更具当前产品型号，得到一段时间内的OK数目，NG数目。\n# 2020-7-13 13:57:47"
        n42 = Index Array(array=w242, index #1=1 ("index"), index #3=6 ("index")) -> (element #1=w238:string, element #2=w237:string, element #3=w245:string)  [unwired: 1 in]
        n43 = Array Subset(array=w242, index=14, length=30) -> (w248:string[])
        n44 = call "Get Main.Parmeters.vi"("Main"=w240, "VariableName"="SelectResultsDataStartDatetime") -> ()  [unwired: 6 in, 8 out]
        n45 = Format Date/Time String(time format string (%c)="%Y-%m-%d %H:%M:%S") -> (date/time string=w260:string)  [unwired: 2 in]
        n46 = Format Date/Time String(time format string (%c)="%Y-%m-%d 00:00:00") -> (date/time string=w228:string)  [unwired: 2 in]
        n47 = Build Array (concatenate)(w238, w237, w245, w248) -> (w241:string[])
        n48 = Index Array(array=w242, index #1=1 ("index"), index #2=6 ("index"), index #3=0 ("index")) -> (element #1=w276:string, element #2=w254:string, element #3=w252:string)
        n49 = Build Array(w276, w254) -> ()  [unwired: 1 out]
        n50 = call <userlib>:"Create Between DateTime.vi"("HaveWhere?"=TRUE, "End DateTime"=w260, "Start DateTime"=w228, "Column Name"=w252) -> ("Between DateTime"=w256:string)  [unwired: 7 in]
        n51 = call <userlib>:"SQL_Select From DB Table.vi"("DB Type"=T2."SQLite", "SelectedColumnsNameList"=w241, "TableName"=w273) -> ("Select SQL CMD"=w263:string)  [unwired: 8 in]
        n52 = Concatenate Strings(w263, w256) -> (w257:string)
        n53 = call-dynamic "SQL Execute.vi"("error in (no error)"=w268, "Command Text"=w257, "HostDB in"=w272) -> ("error out"=w267:errorcluster, "Table Control"=w229:string[][], "HostDB out"=w271:refnum<class "SQLite.lvclass">)  [unwired: 4 in, 2 out]
        n54 = Array Size(array=w229) -> (size(s)=w236:i32[])
        n55 = Index Array(array=w236, index=0) -> (element=w232:i32)
        n56 = Greater Or Equal?(x=w232, y=w233) -> (x >= y?=w234:bool)
        n57 = Subtract(x=w232, y=50) -> (x-y=w230:i32)
        n58 = call <vilib>:"Add State(s) to Queue__jki_lib_state_machine.vi"("State(s) in Front (\"\")"=w262, "State(s) in (\"\")"=w257) -> ("States Out"=w264:string)  [unwired: 13 in]
        n59 = case shown="True" w234 {
          tunnel: w229 -> [w281 w285]
          tunnel: w233 -> [_ w284]
          tunnel: w230 -> [_ w283]
          tunnel: [w281 w282] -> w225
          frame False {
          }
          frame True {
            n60 = Array Subset(array=w285, index (row)=w283, length (row)=w284) -> (w282:string[][])  [unwired: 2 in]
          }
        }
        "Table Control" <- w225
        n61 = Array Size(array=w225) -> (size(s)=w226:i32[])
        n62 = Index Array(array=w226, index=0) -> (element=w224:i32)
        n63 = for {
          N: w224 -> [_]
          tunnel: [w278] -> w223 mode=indexing
          i -> [w280]
          n64 = Increment(x=w280) -> (x+1=w279:i32)
          n65 = Number To Decimal String(number=w279) -> (decimal integer string=w278:string)  [unwired: 1 in]
        }
        "Row Num List" <- w223
        n66 = call <vilib>:"Add State(s) to Queue__jki_lib_state_machine.vi"("State(s) in (\"\")"=w269) -> ("States Out"=w270:string)  [unwired: 14 in]
        n67 = call <vilib>:"Add State(s) to Queue__jki_lib_state_machine.vi"("State(s) in (\"\")"=w265, "State(s) at Back (\"\")"=w264) -> ("States Out"=w266:string)  [unwired: 13 in]
      }
      frame "Close" {
        n68 = call-dynamic "Close Connection.vi"("error in (no error)"=w287, "HostDB in"=w289) -> ("error out"=w286:errorcluster, "HostDB out"=w288:refnum<class "SQLite.lvclass">)  [unwired: 8 in]
      }
    }
  }
  "error out" <- w4
  "CMD" <- w3
  n69 = Random Number (0-1)() -> (number: 0 to 1=→"number (0 to 1)":dbl)
